vi "verifyEnemyTarget.vi"(8 "error in (no error)":errorcluster, 9 "GoalWidth/2":dbl format="%#_13g", 10 "EnemtyTargetInModlue":dbl format="%#_13g", 11 "DefendGoalTactic in":refnum<class "DefendGoalTactic.lvclass">) -> (0 "error out":errorcluster, 2 "TargetInsideGoal":bool, 3 "DefendGoalTactic out":refnum<class "DefendGoalTactic.lvclass">)   [LabVIEW 2024, in "DefendGoalTactic.lvclass"]
uses:
  DefendGoalTactic.lvclass
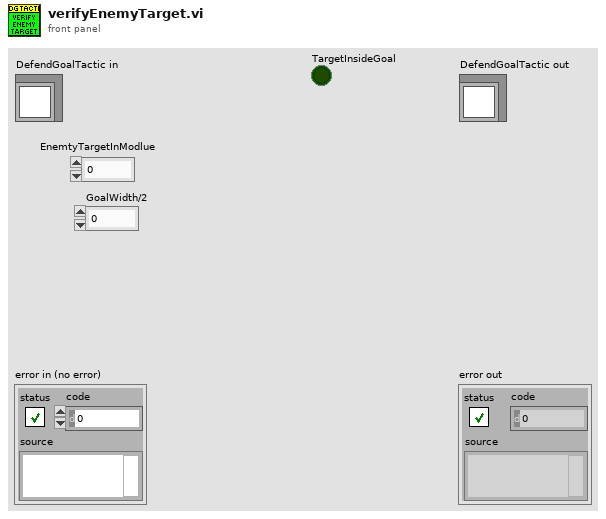
[diagram p1: front panel]
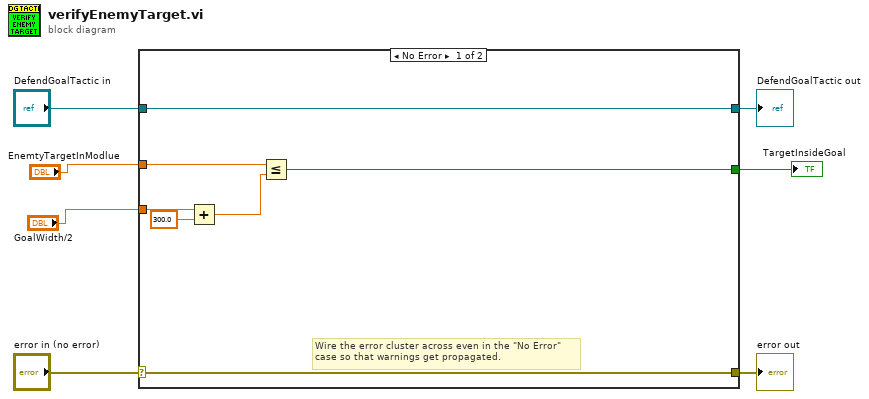
[diagram p0: block diagram]
diagram:
  n1 = case shown="No Error" "error in (no error)" {
    selector: "error in (no error)" -> [w13 w16]
    tunnel: [w13 w16] -> w6
    tunnel: [w14 w15] -> w4
    tunnel: "DefendGoalTactic in" -> [w14 w15]
    tunnel: "GoalWidth/2" -> [w12 _]
    tunnel: "EnemtyTargetInModlue" -> [w10 _]
    tunnel: [w8 _] -> w1
    frame No Error {
      # "Wire the error cluster across even in the \"No Error\"\ncase so that warnings get propagated."
      n2 = Add(x=w12, y=300.0) -> (x+y=w9:dbl)
      n3 = Less Or Equal?(x=w10, y=w9) -> (x <= y?=w8:bool)
    }
    frame Error {
    }
  }
  "error out" <- w6
  "DefendGoalTactic out" <- w4
  "TargetInsideGoal" <- w1
